vi "MoveCoordTemplate.vi"(7 "MoveAction":enum16{"ToTemp", "ToData"}(ring), 8 "error in (no error)":errorcluster, 9 "Paths":path[](array[path]), 10 "Project":string, 11 "Root In":path) -> (0 "error out":errorcluster, 3 "Root Out":path)   [LabVIEW 2019]
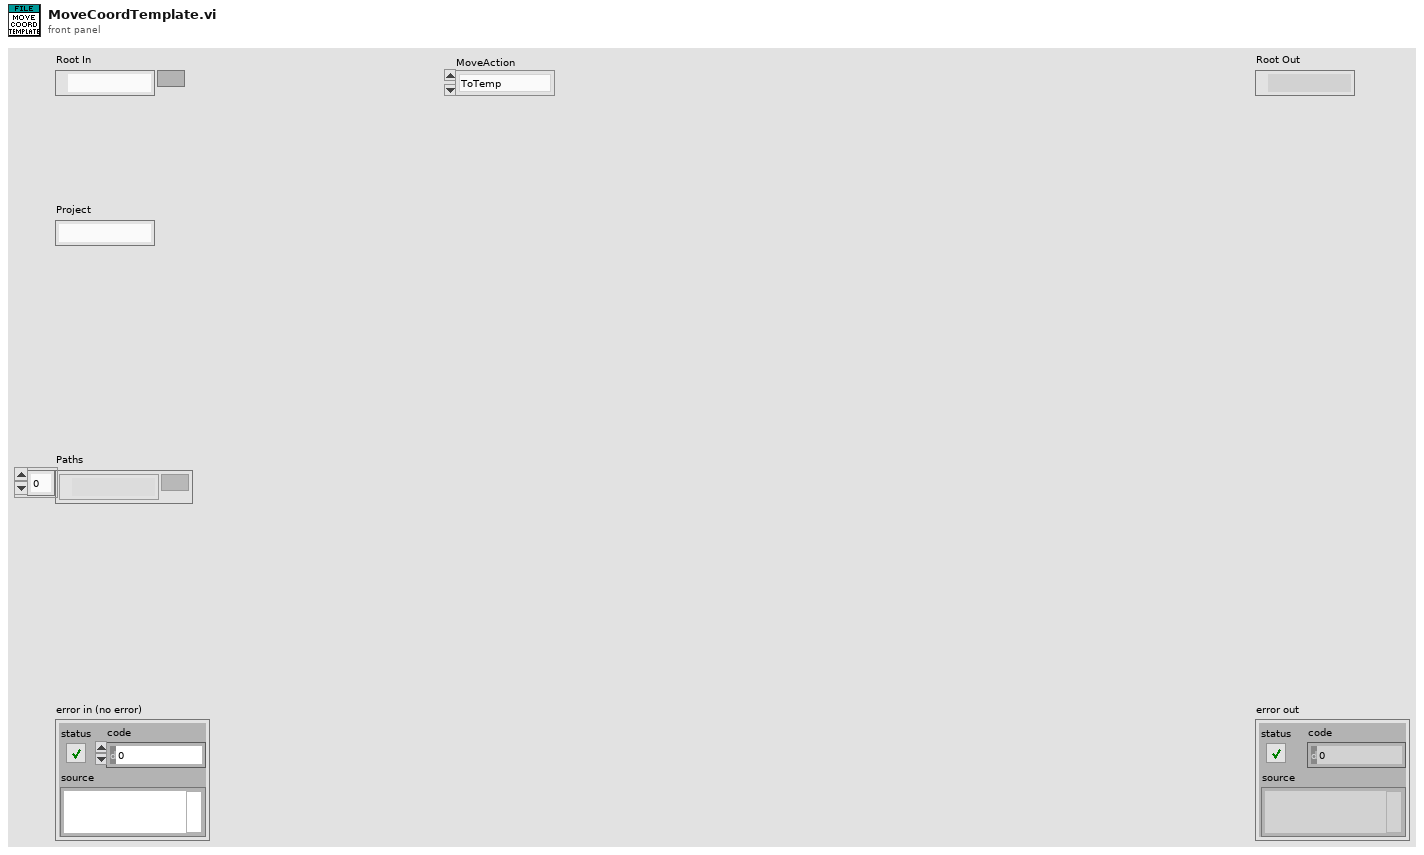
[diagram p1: front panel]
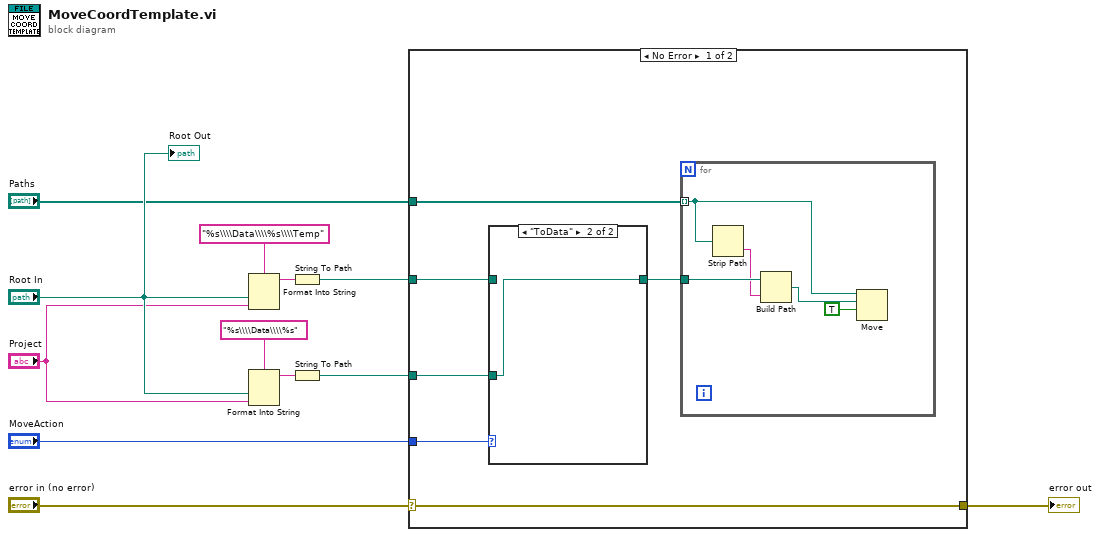
[diagram p0: block diagram]
diagram:
  n1 = Format Into String(format string="%s\\\\Data\\\\%s\\\\Temp", "Root In", "Project") -> (resulting string=w10:string)  [unwired: 2 in, 1 out]
  n2 = Format Into String(format string="%s\\\\Data\\\\%s", "Root In", "Project") -> (resulting string=w9:string)  [unwired: 2 in, 1 out]
  n3 = String To Path(string=w10) -> (path=w5:path)
  n4 = String To Path(string=w9) -> (path=w4:path)
  n5 = case shown="No Error" "error in (no error)" {
    selector: "error in (no error)" -> [w18 w26]
    tunnel: [w18 w26] -> w1
    tunnel: w5 -> [w15 _]
    tunnel: w4 -> [w13 _]
    tunnel: "Paths" -> [w17 _]
    tunnel: "MoveAction" -> [w16 _]
    frame No Error {
      n6 = case shown="\"ToData\"" w16 {
        tunnel: w15 -> [w19 _]
        tunnel: [w19 w20] -> w14
        tunnel: w13 -> [_ w20]
        frame "ToTemp", Default {
        }
        frame "ToData" {
        }
      }
      n7 = for {
        tunnel: w14 -> [w24]
        tunnel: w17 -> [w25] mode=indexing
        n8 = Strip Path(path=w25) -> (name=w23:string)  [unwired: 1 out]
        n9 = Build Path(base path=w24, name or relative path=w23) -> (appended path=w22:path)
        n10 = Move(source path=w25, 9:TRUE ("overwrite (F)"), 10:w22) -> ()  [unwired: 2 in, 3 out]
      }
    }
    frame Error {
    }
  }
  "error out" <- w1
  "Root Out" <- "Root In"
